vi "create box and whisker plot.vi"(1 "Array In":dbl[](array[numeric])) -> (0 "Box and whisker plot":cluster{dbl, dbl, dbl, dbl, dbl}(slide)={0.8333333333333333, 2.083333333333333, 5.059523809523809, 8.095238095238095, 10.0} scale=0.0..10.0)   [LabVIEW 2009]
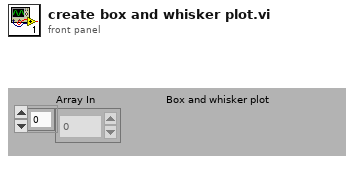
[diagram p1: front panel]
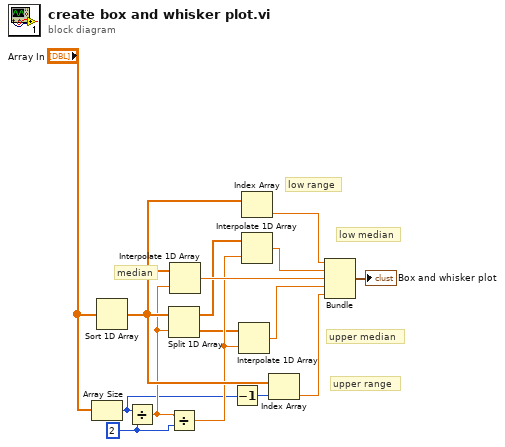
[diagram p0: block diagram]
diagram:
  w7 = 2 ("y")
  # "upper range"
  # "upper median"
  # "median"
  # "low median"
  # "low range"
  n1 = Array Size(array="Array In") -> (size(s)=w5:i32)
  n2 = Sort 1D Array(array="Array In") -> (sorted array=w9:dbl[])
  n3 = Divide(x=w5, y=w7) -> (x/y=w6:dbl)
  n4 = Split 1D Array(array=w9, index=w6) -> (first subarray=w3:dbl[], second subarray=w4:dbl[])
  n5 = Divide(x=w6, y=w7) -> (x/y=w8:dbl)
  n6 = Interpolate 1D Array(1:w6, 2:w9) -> (0:w12:dbl)
  n7 = Decrement(x=w5) -> (x-1=w1:i32)
  n8 = Interpolate 1D Array(1:w8, 2:w4) -> (0:w14:dbl)
  n9 = Index Array(array=w9) -> (element=w10:dbl)  [unwired: 1 in]
  n10 = Interpolate 1D Array(1:w8, 2:w3) -> (0:w11:dbl)
  n11 = Index Array(array=w9, index=w1) -> (element=w13:dbl)
  n12 = Bundle(w10, w11, w12, w14, w13) -> (→"Box and whisker plot":cluster{dbl, dbl, dbl, dbl, dbl})  [unwired: 1 in]
